vi "_Test_RDB Receive Points.vi"() -> ()   [LabVIEW 2023]
uses:
  RDB/RDB.lvlib
panel:
  out "signal data":dbl[](array[numeric]) format="%.2f"
  out "number":i32[](array[numeric])
  out "offset past match":i32
  in  "String":string
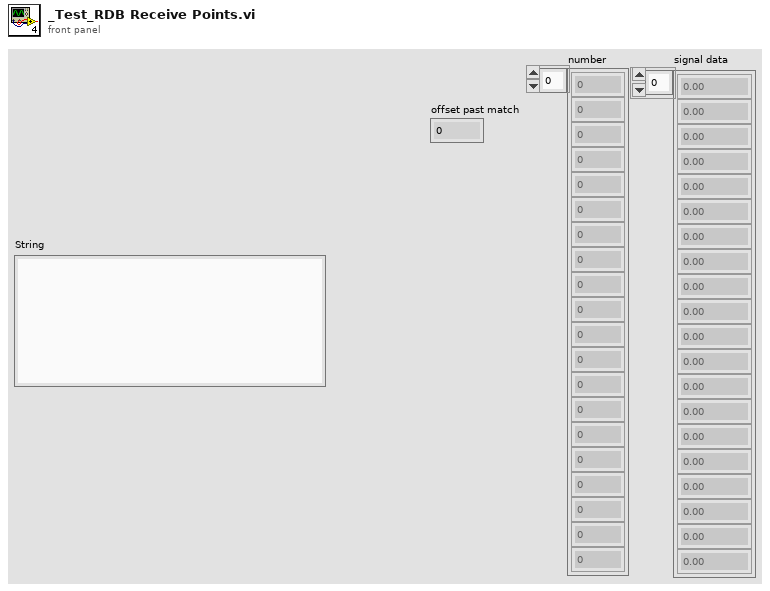
[diagram p1: front panel]
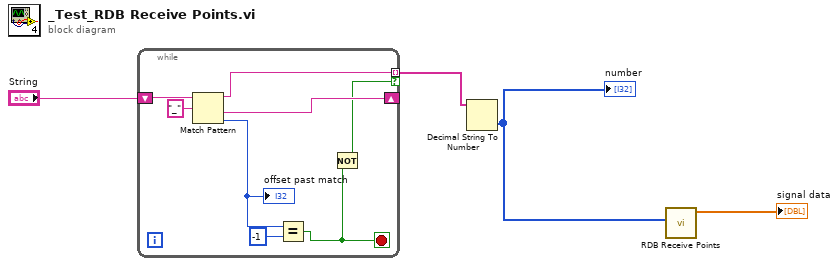
[diagram p0: block diagram]
diagram:
  n1 = while {
    shift-right: [w10] -> _
    shift-left: "String" -> [w12]
    tunnel: [w11] -> w3 mode=indexing if=w5
    stop <- w6 stop-if-true
    n2 = Match Pattern(string=w12, regular expression="_") -> (before substring=w11:string, after substring=w10:string, offset past match=w8:i32)  [unwired: 1 in, 1 out]
    "offset past match" <- w8
    n3 = Equal?(x=w8, y=-1) -> (x = y?=w6:bool)
    n4 = Not(x=w6) -> (.not. x?=w5:bool)
  }
  n5 = Decimal String To Number(string=w3) -> (number=w2:i32[])  [unwired: 2 in, 1 out]
  "number" <- w2
  n6 = call "RDB Receive Points.vi"("Data"=w2) -> ("signal data"=→"signal data":dbl[])  [unwired: 10 in]
